vi "GenUniqueName.vi"() -> (0 "Uniquename":string)   [LabVIEW 2019, in "CAN-NI.lvlib" / "CAN-NI.lvclass"]
uses:
  CAN-NI.lvclass
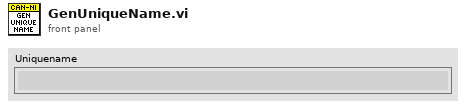
[diagram p1: front panel]
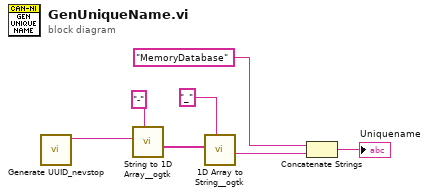
[diagram p0: block diagram]
diagram:
  n1 = call <userlib>:"Generate UUID_nevstop.vi"() -> ("UUID"=w1:string)  [unwired: 11 in]
  n2 = call <userlib>:"String to 1D Array__ogtk.vi"("delimiter (Tab)"="-", "string"=w1) -> ("Array of Strings"=w3:string[])  [unwired: 9 in]
  n3 = call <userlib>:"1D Array to String__ogtk.vi"("delimiter (Tab)"="_", "Array of Strings"=w3) -> ("delimited string"=w4:string)  [unwired: 9 in]
  n4 = Concatenate Strings("MemoryDatabase" ("string"), w4) -> (→"Uniquename":string)
